vi "Configure LabVIEW Build.vi"(8 "error in (no error)":errorcluster, 10 "JSON string":string) -> (0 "error out":errorcluster, 3 "EXE Build out":refnum<class "LabVIEW Build.lvclass">)   [LabVIEW 2014, in "LabVIEW Build.lvclass"]
uses:
  LabVIEW Build.lvclass
  Shared/Controls/LabVIEW Build - STYP.ctl
  Classes/Job/Job.lvclass/Job.ctl
  LabVIEW Build.lvclass/LabVIEW Build.ctl
  Classes/Job/Write Executor Number.vi
  Classes/Job/Write WorkSpace Path.vi
  Write Auto Version Increment_.vi
  Write Build Spec.vi
  Write Project Path.vi
  Write Target.vi
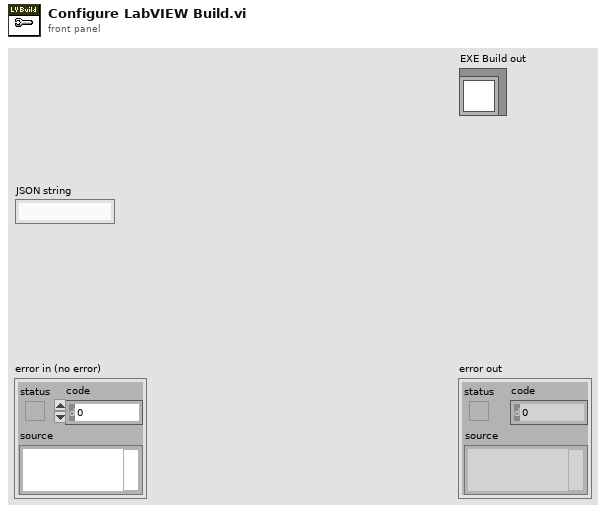
[diagram p1: front panel]
types:
  T1 = typedef "LabVIEW Build - STYP.ctl" = cluster{"Executor_Number":string, "Workspace_Path":string, "Build_Spec":string, "Target":string, "Project_Path":string, "Auto_Version_Increment":bool}
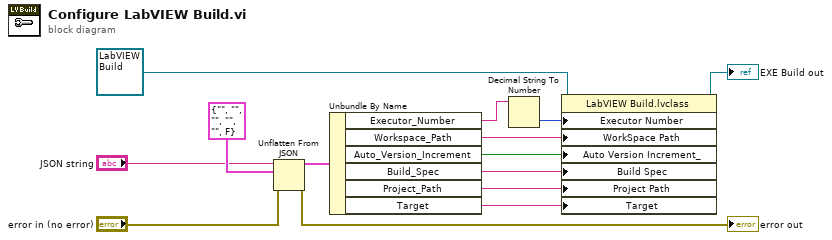
[diagram p0: block diagram]
diagram:
  n1 = Unflatten From JSON(JSON string="JSON string", type and defaults=T1 {"Executor_Number"="", "Workspace_Path"="", "Build_Spec"="", "Target"="", "Project_Path"="", "Auto_Version_Increment"=FALSE} ("EXE_Build"), error in (no error)="error in (no error)") -> (value=w10:T1, error out=→"error out":errorcluster)  [unwired: 4 in]
  n2 = Unbundle By Name(w10) -> ("Executor_Number"=w13:string, "Workspace_Path"=w6:string, "Auto_Version_Increment"=w4:bool, "Build_Spec"=w3:string, "Project_Path"=w2:string, "Target"=w1:string)
  n3 = Decimal String To Number(string=w13) -> (number=w5:i32)  [unwired: 2 in, 1 out]
  n4 = property class="LabVIEW Build.lvclass"(reference=refnum<class "LabVIEW Build.lvclass"> refnum ("EXE Build in"), "Executor Number"=w5, "WorkSpace Path"=w6, "Auto Version Increment_"=w4, "Build Spec"=w3, "Project Path"=w2, "Target"=w1) -> (reference out=→"EXE Build out":refnum<class "LabVIEW Build.lvclass">)  [unwired: 1 in, 1 out]
